vi "Main.vi"() -> ()   [LabVIEW 2025]
doc: "Use this template to build a simple state machine design pattern. Each state executes code and determines which state to transition to."
uses:
  <vilib>/Utility/miscctls.llb/LVPoint32TypeDef.ctl
  controls/State.ctl
  controls/Data.ctl
  multi.ctl
  controls/playerstatus.ctl
panel:
  in  "Boolean":bool
  out "lose":bool=TRUE
  out "win":bool=TRUE
  out "Coords":T1
  out "main tab":T2(tab) caption="Tab Control"
  in  "stop":bool
  in  "Edit entry":bool
  in  "multi entry":bool
  in  "sing entry":bool
  in  "Sp.AI entry":bool
  in  "Countdown entry":bool
  in  "Classic entry":bool
  in  "go back (sel)":bool
  in  "Size (<=25, square)":i32=3 min=3 max=25 step=1
  in  "Layers (<=64)":i32=1 min=1 max=64 step=1
  in  "Toggle barrier":bool
  in  "mapgen sw":bool
  out "multi player status":cluster{"score":i32, "name":string}[](array[cluster])
  out "score":dbl
  out "flag wrong":i32
  out "flag correct":i32
  in  "reset button":bool
  in  "page up":bool
  out "pagenum":i32
  in  "page down":bool
  out "timer":timestamp format="%<%H:%M:%S%3u>T"
  in  "go back (ingame)":bool
  out "2D Picture":picture
  in  "clean\nall\nmulti\nplayer\nand\nleave":bool
  in  "LEAVE":bool
  in  "HOST":bool
  in  "READY":bool
  out "multi player status":cluster{"score":i32, "name":string}[](array[cluster])
  out "timestart":dbl format="%_19f"
  # "map select"
  # "auto gen"
  # "load file"
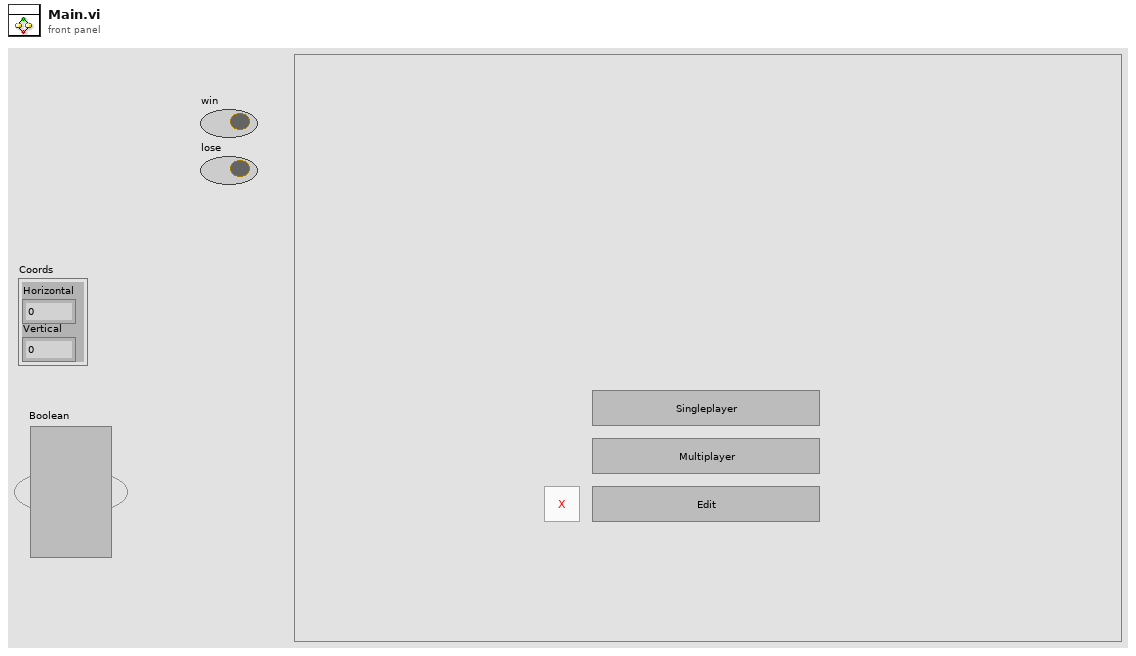
[diagram p1: front panel]
types:
  T1 = typedef "LVPoint32TypeDef.ctl" = cluster{"Horizontal":i32, "Vertical":i32}
  T2 = enum32{"menu", "select page", "sing", "multi", "multi setting"}
  T3 = typedef "Data.ctl" = cluster{"barrier":bool, "username":string, "Numeric <Replace Me>":dbl, "player mode":u16, "mode":u16, "layers":i32, "size":i32, "sec":i32}
  T4 = typedef "State.ctl" = enum16{"Initialize", "Menu", "select map", "ingame", "multi(abanden)", "edit", "Exit"}
  T5 = enum8{"Enabled", "Disabled", "Disabled and Grayed Out"}
  T6 = typedef "playerstatus.ctl" = cluster{"correct flag":i32, "wrong flag":i32, "username":string, "status":u16}
  T7 = typedef "multi.ctl" = cluster{"Array":i8[][][], "player":T6[], "layer":i32, "size":i32, "mode":u16, "sec":i32, "minecount":i32}
  T8 = cluster{"left":i16, "top":i16, "right":i16, "bottom":i16}
  T9 = typedef "LVDateTimeRec.ctl" = cluster{"fractional second":dbl, "second":i32, "minute":i32, "hour":i32, "day of month":i32, "month":i32, "year":i32, "day of week":i32, "day of year":i32, "DST":i32}
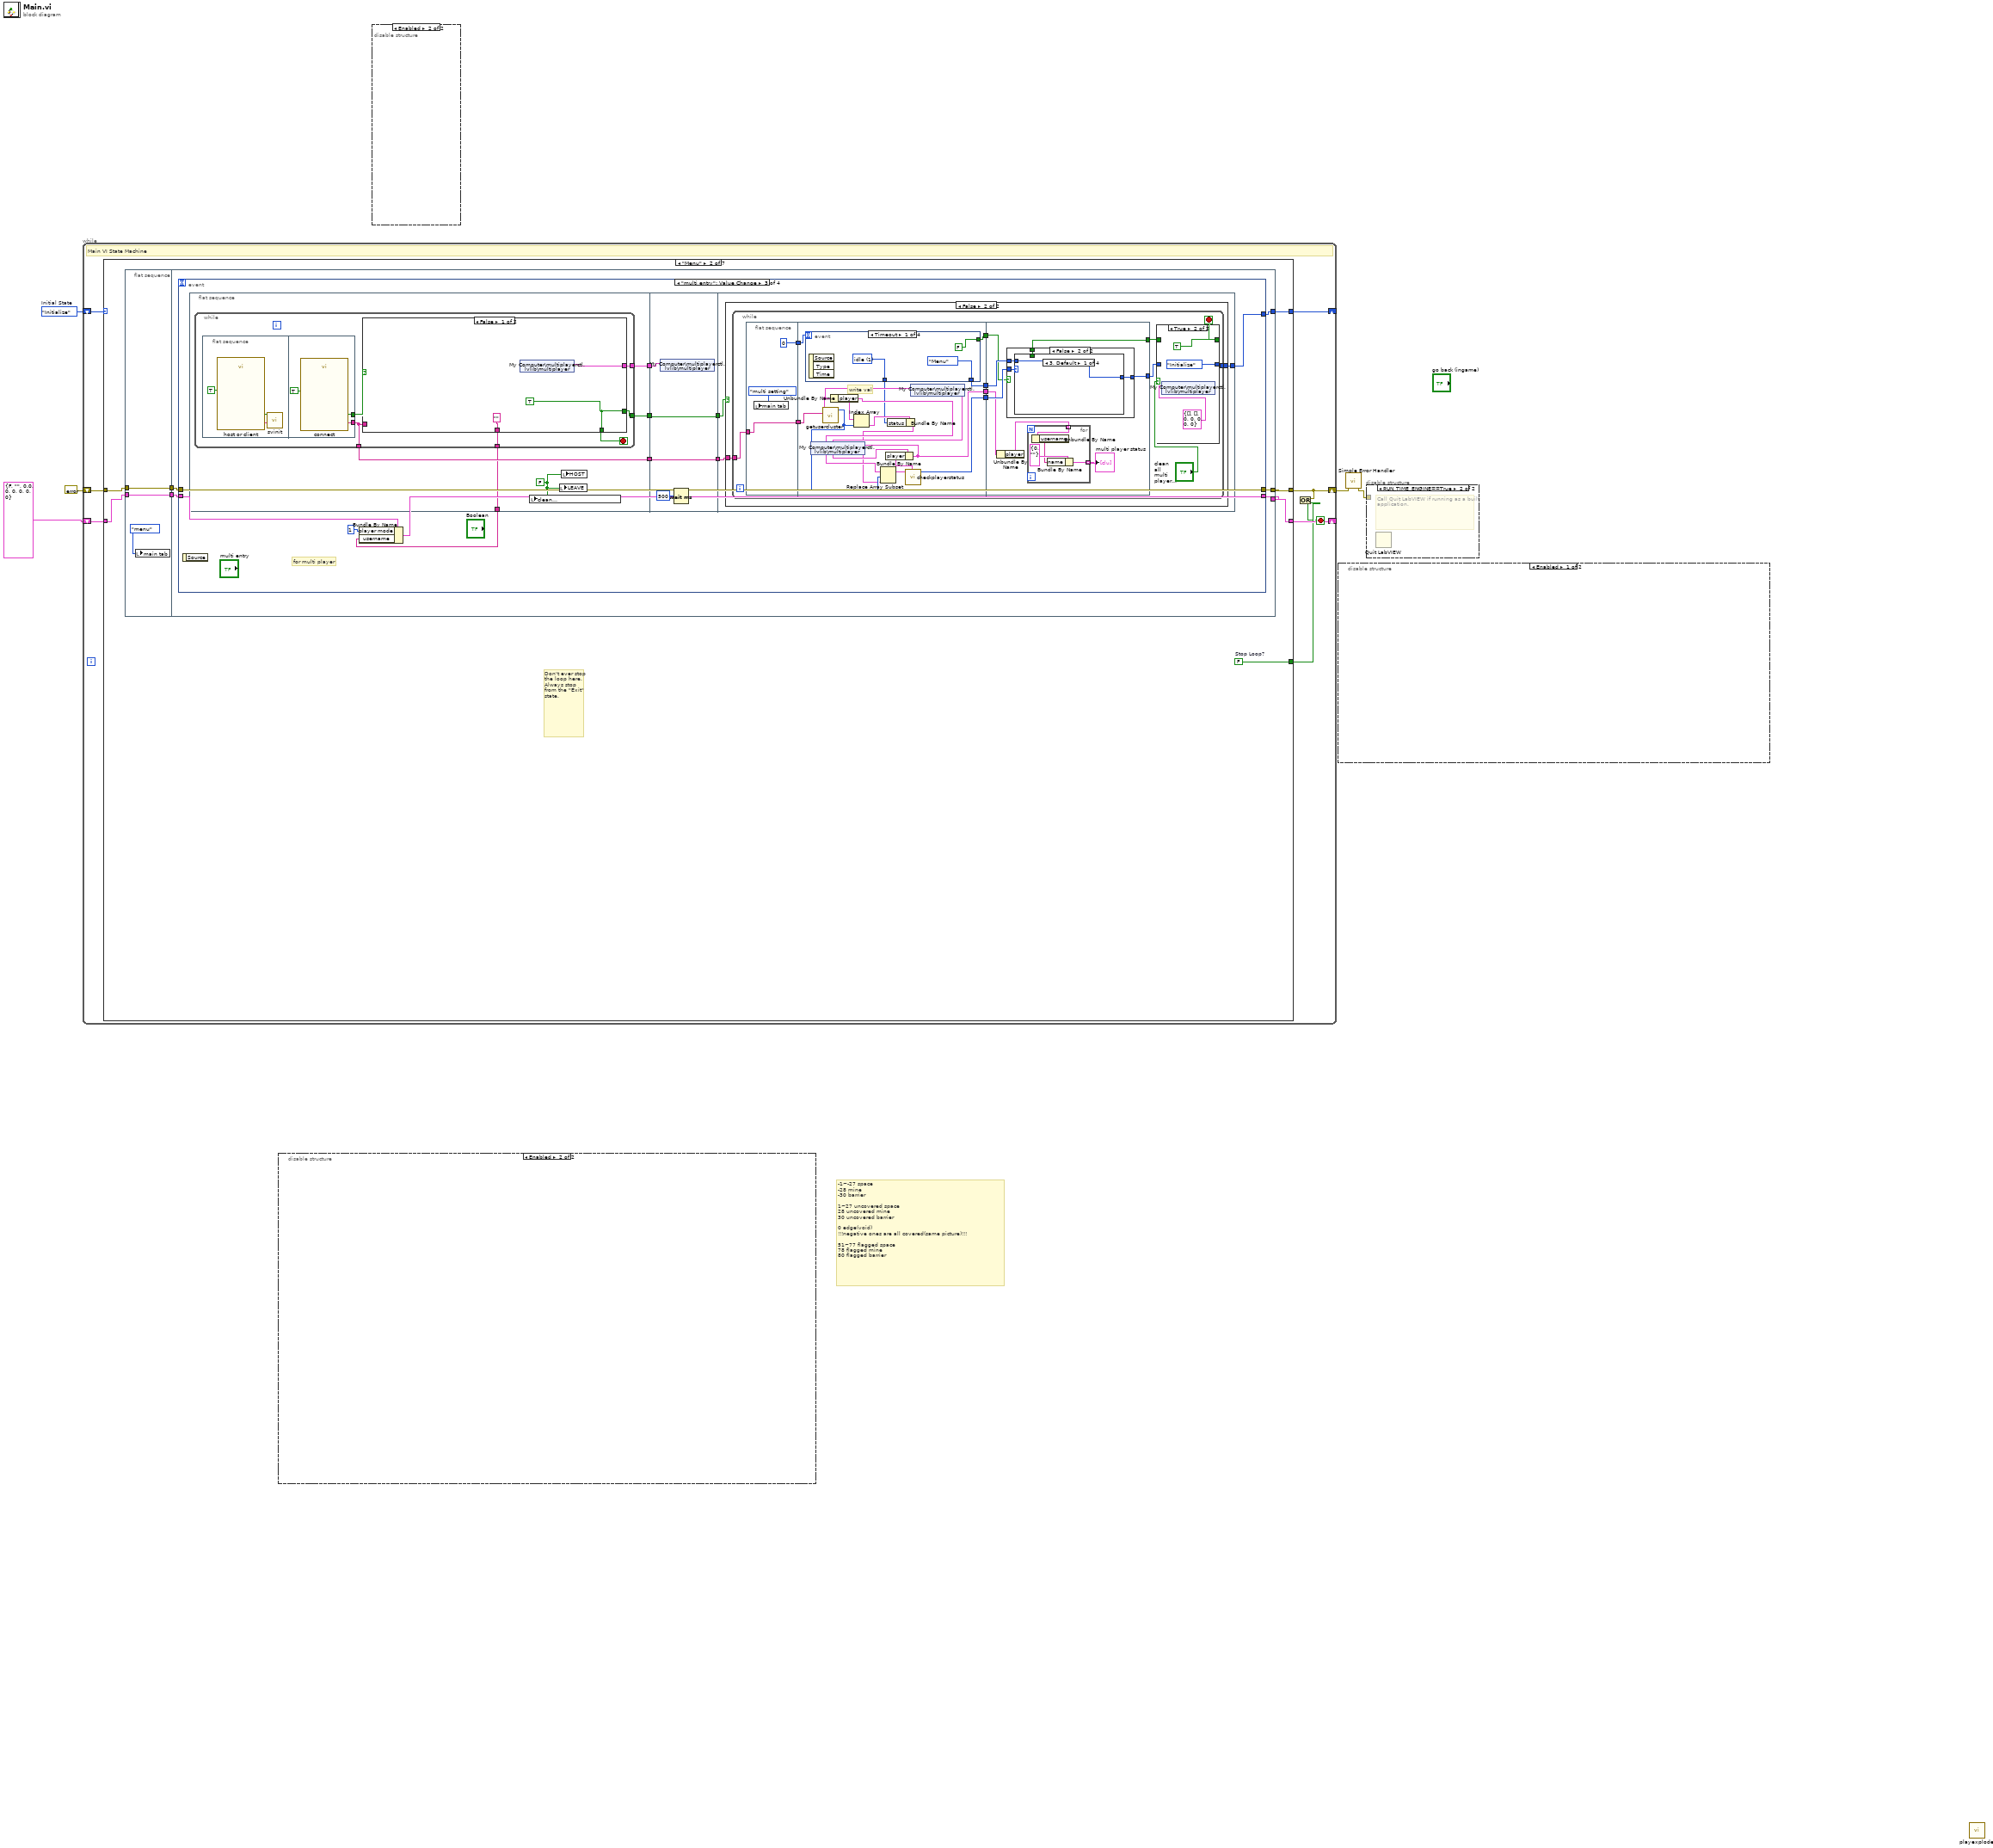
[diagram p0: block diagram]
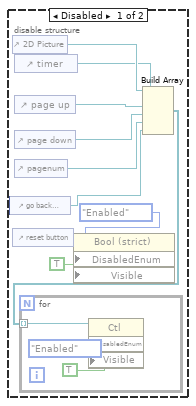
[diagram p3: hidden frame]
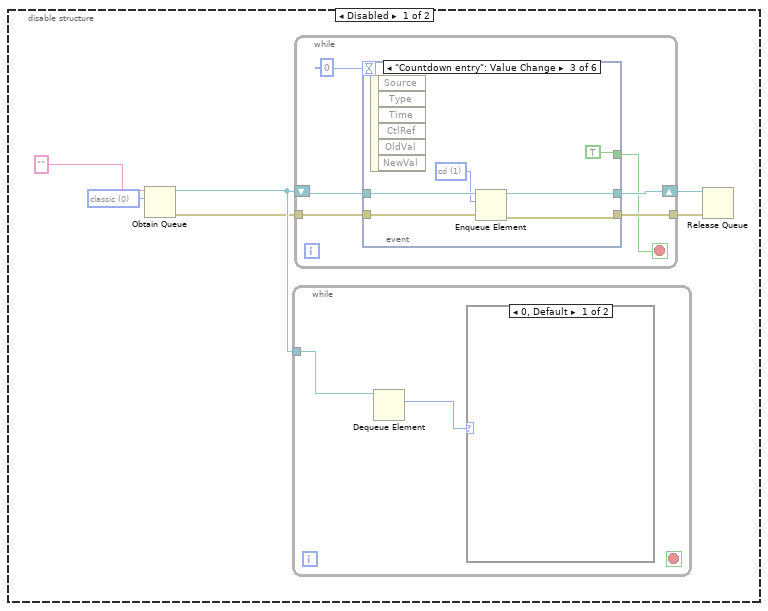
[diagram p4: hidden frame]
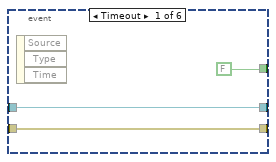
[diagram p6: hidden frame]
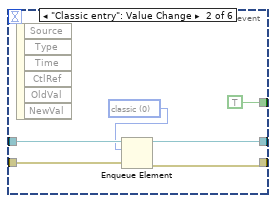
[diagram p7: hidden frame]
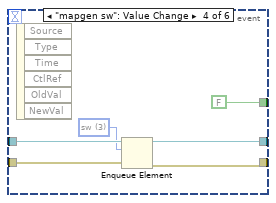
[diagram p8: hidden frame]
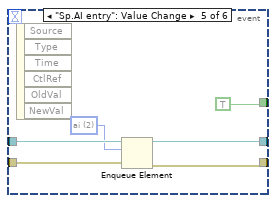
[diagram p9: hidden frame]
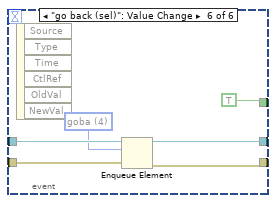
[diagram p10: hidden frame]
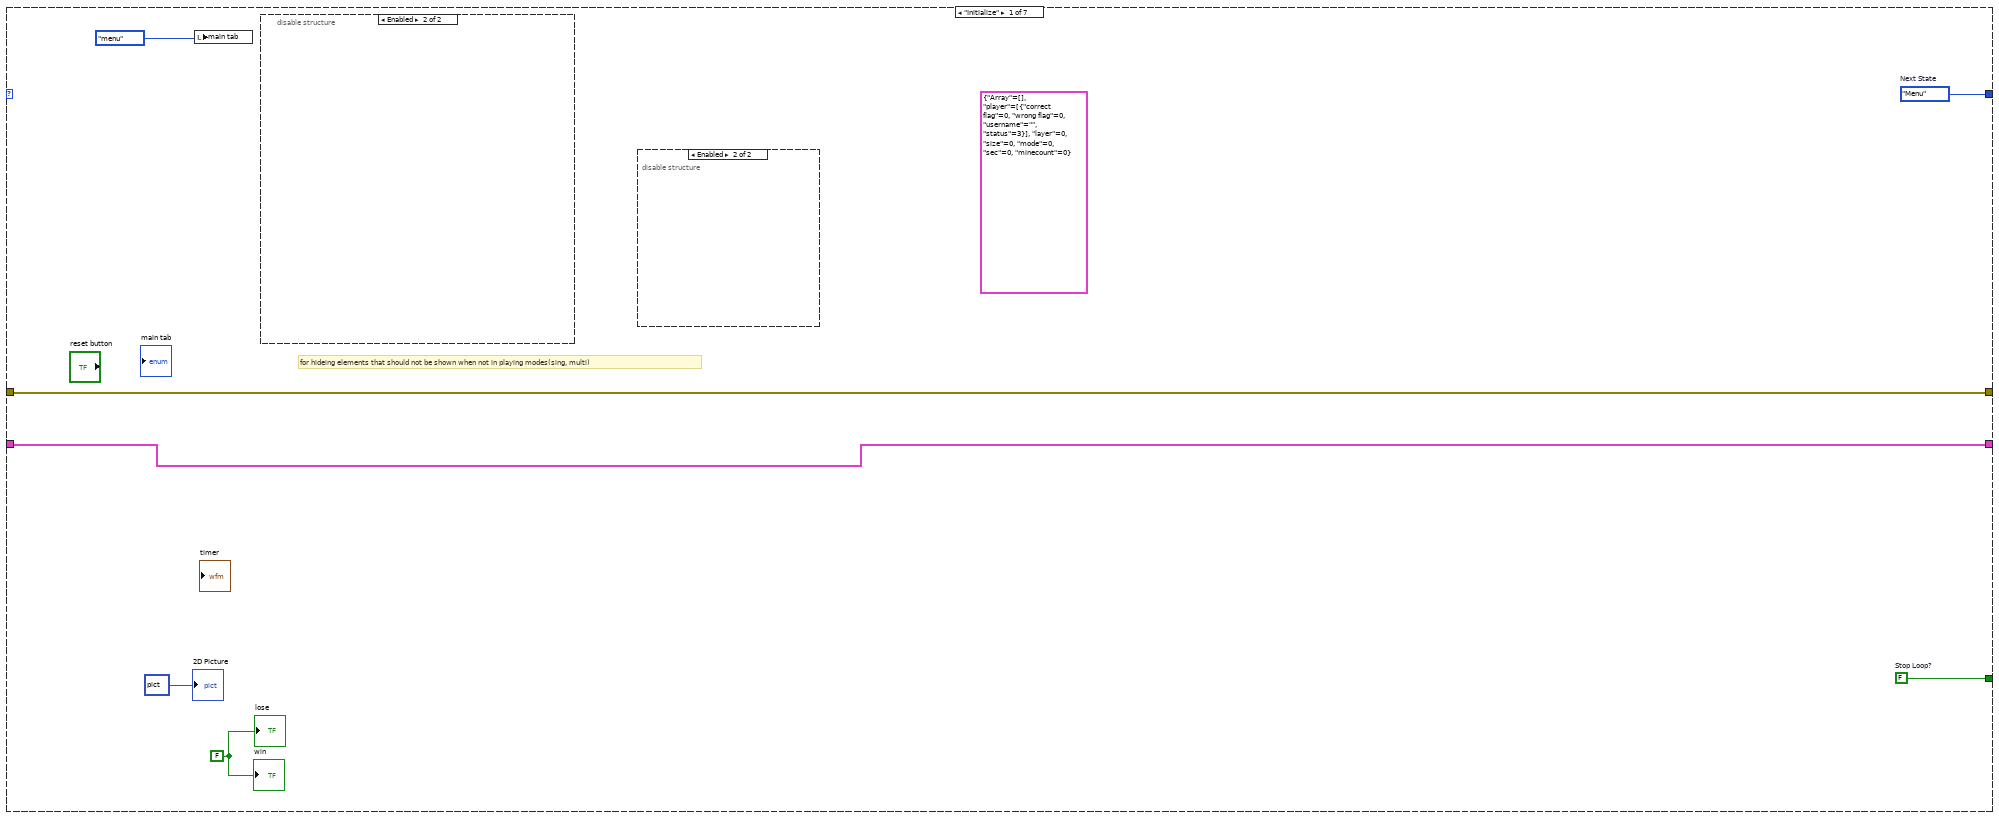
[diagram p12: hidden frame]
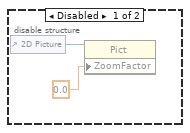
[diagram p13: hidden frame]
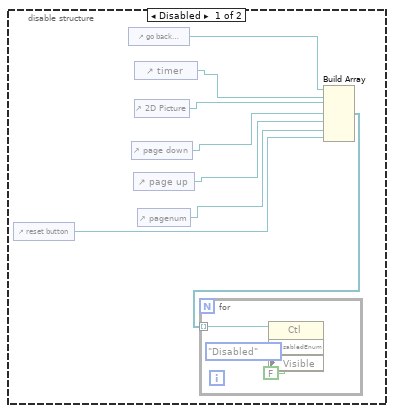
[diagram p14: hidden frame]
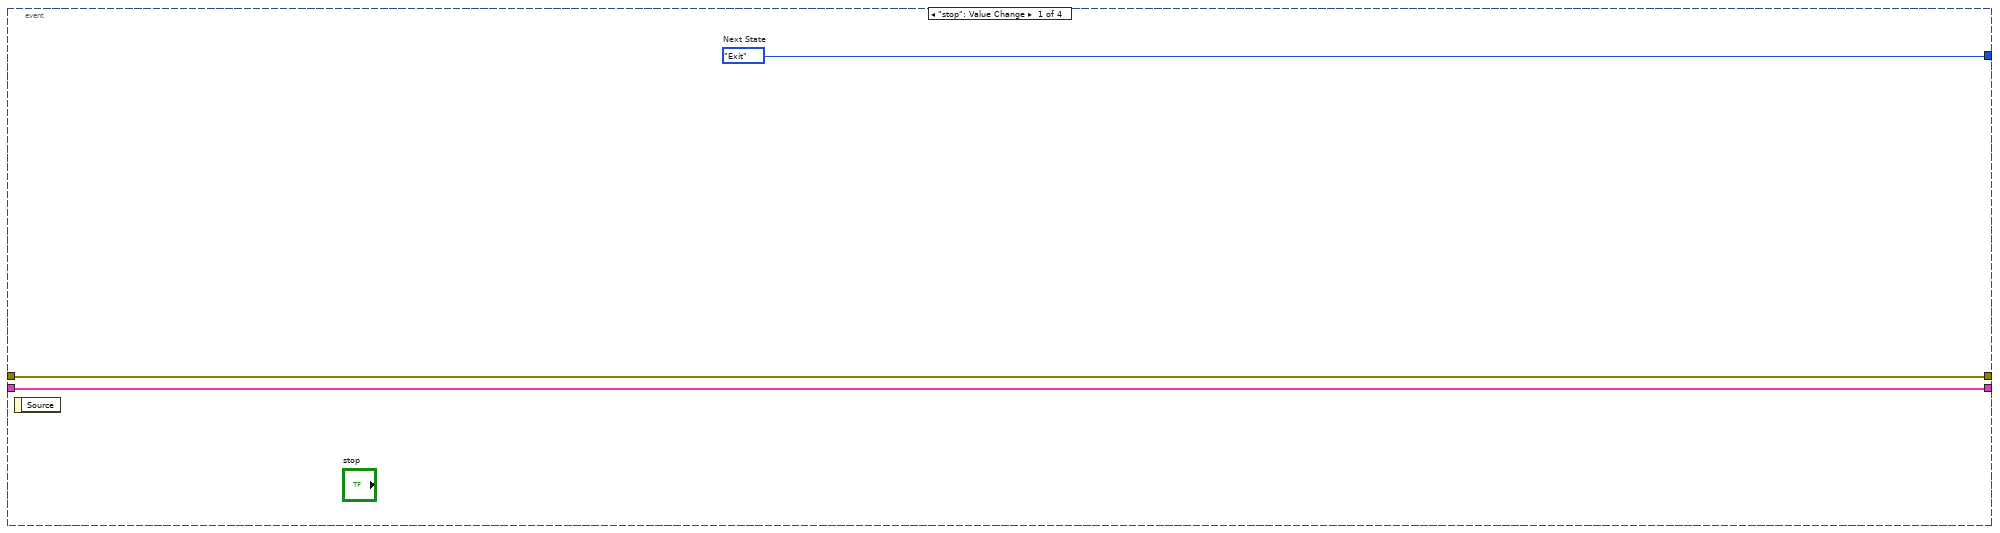
[diagram p15: hidden frame]
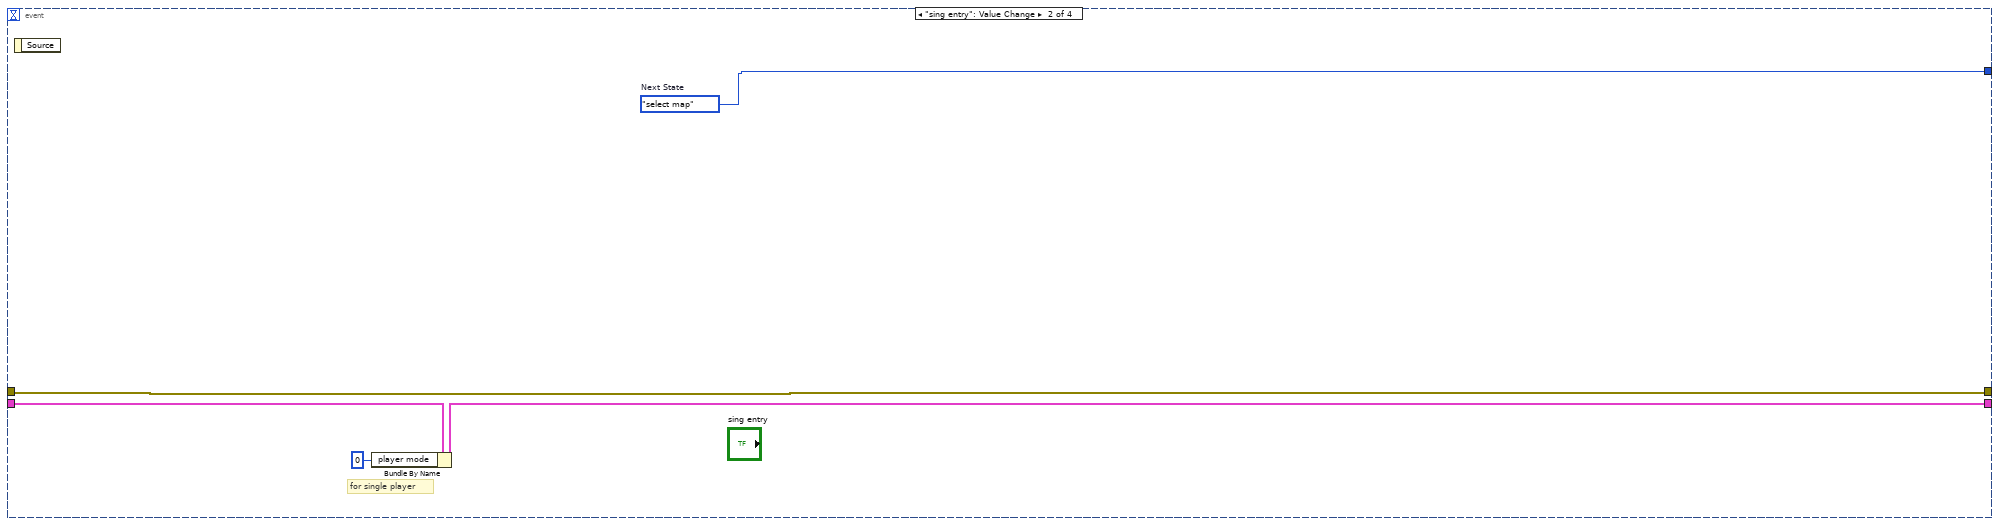
[diagram p16: hidden frame]
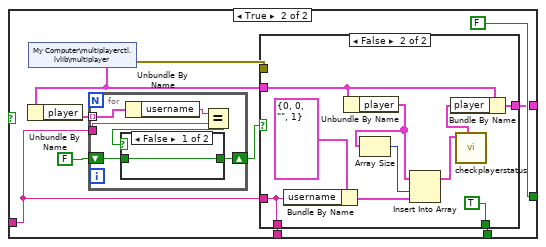
[diagram p17: hidden frame]
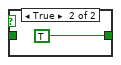
[diagram p18: hidden frame]
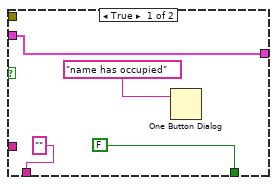
[diagram p19: hidden frame]
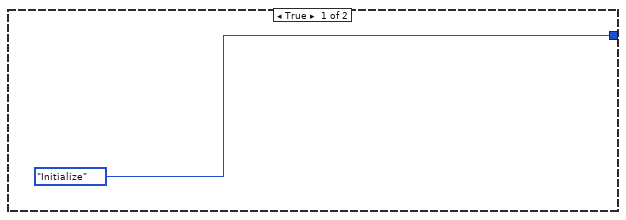
[diagram p20: hidden frame]
diagram:
  w1 = State."Initialize"  # Initial State
  # "-1~-27 space\n-28 mine\n-30 barrier\n\n1~27 uncovered space\n28 uncovered mine\n30 uncovered barrier\n\n0 edge(void)\n!!!negative ones are all covered(same picture)!!!\n\n51~77 flagged space\n78 flagged mine\n80 flagged barrier"
  n1 = while {
    shift-right: [w12] -> _
    shift-left: T3 {"barrier"=FALSE, "username"="", "Numeric <Replace Me>"=0.0, "player mode"=0, "mode"=0, "layers"=0, "size"=0, "sec"=0} ("Data") -> [w13]
    shift-right: [w8] -> w4
    shift-left: errorcluster {"status"=FALSE, "code"=0, "source"=""} ("error constant") -> [w11]
    shift-right: [w6] -> _
    shift-left: w1 -> [w7]
    stop <- w9 stop-if-true
    # "Main VI State Machine"
    n2 = case shown="\"Menu\"" w7 {
      selector: w7 -> [_ _ w204 _ _ _ _]
      tunnel: [w20 w41 w204 w209 w281 w754 w758] -> w6
      tunnel: [w19 w40 TRUE ("Stop Loop?") FALSE ("Stop Loop?") FALSE ("Stop Loop?") FALSE ("Stop Loop?") w756] -> w10
      tunnel: w13 -> [w17 w39 w207 w211 w274 w752 w757]
      tunnel: [w17 w38 w207 w212 w273 w752 w757] -> w12
      tunnel: w11 -> [w18 w37 w206 w214 w285 w751 w755]
      tunnel: [w18 w36 w206 w214 w285 w751 w755] -> w8
      frame "Initialize" {
        (unwired) T7 {"Array"=[], "player"=[{"correct flag"=0, "wrong flag"=0, "username"="", "status"=3}], "layer"=0, "size"=0, "mode"=0, "sec"=0, "minecount"=0} ("multiplayer")
        w16 = FALSE ("lose")
        w19 = FALSE  # Stop Loop?
        w20 = State."Menu"  # Next State
        # "for hideing elements that should not be shown when not in playing modes(sing, multi)"
        # "Initialize - Initialize the application."
        n3 = local write "main tab"(T2."menu" ("main tab")) -> ()
        n4 = disable-structure shown="Enabled" {
          frame Disabled {
            n5 = control-ref of="reset button"() -> (w24:refnum<vi>)
            n6 = control-ref of="go back (ingame)"() -> (w23:refnum<vi>)
            n7 = control-ref of="page down"() -> (w27:refnum<vi>)
            n8 = control-ref of="page up"() -> (w26:refnum<vi>)
            n9 = control-ref of="timer"() -> (w29:refnum<vi>)
            n10 = control-ref of="2D Picture"() -> (w28:refnum<vi>)
            n11 = control-ref of="pagenum"() -> (w25:refnum<vi>)
            n12 = Build Array(w23, w29, w28, w27, w26, w25, w24) -> (w30:refnum<vi>[])
            n13 = for {
              tunnel: w30 -> [w31] mode=indexing
              n14 = property on="Property Node" class="Ctl"(reference=w31, "DisabledEnum"=T5."Disabled" ("Disabled"), "Visible"=FALSE) -> ()  [unwired: 1 in, 2 out]
            }
          }
          frame Enabled {
          }
        }
        n15 = disable-structure shown="Enabled" {
          frame Disabled {
            n16 = control-ref of="2D Picture"() -> (w22:refnum<vi>)
            n17 = property on="Property Node" class="Pict"(reference=w22, "ZoomFactor"=sgl 0.0 ("Zoom Factor")) -> ()  [unwired: 1 in, 2 out]
          }
          frame Enabled {
          }
        }
        "win" <- w16
        "lose" <- w16
        "2D Picture" <- picture data[5B] ("2D Picture")
      }
      frame "Menu" {
        w40 = FALSE  # Stop Loop?
        # "Don't ever stop the loop here. Always stop from the \"Exit\" state."
        n18 = flat-sequence {
          tunnel: w37 -> [w43]
          tunnel: w39 -> [w44]
          tunnel: [w44] -> w35
          tunnel: [w43] -> w34
          tunnel: [w49] -> w41
          tunnel: [w45] -> w38
          tunnel: [w46] -> w36
          tunnel: w35 -> [w48]
          tunnel: w34 -> [w47]
          frame #0 {
            n19 = local write "main tab"(T2."menu" ("main tab")) -> ()
          }
          frame #1 {
            n20 = event shown="[2] \"multi entry\": Value Change" {
              selector: _ -> [_ _ _ _]
              dyn-events: _ -> [_ _ _ _]
              timeout: _ -> [_ _ _ _]
              tunnel: [w52 w56 w64 w201] -> w49
              tunnel: w48 -> [w51 w55 w66 w203]
              tunnel: [w51 w53 w65 w203] -> w45
              tunnel: w47 -> [w50 w57 w68 w202]
              tunnel: [w50 w57 w68 w202] -> w46
              event "stop": Value Change {
                w52 = State."Exit"  # Next State
                n21 = event-data() -> ()  [unwired: 1 in, 1 out]
              }
              event "sing entry": Value Change {
                w56 = State."select map"  # Next State
                # "for single player"
                n22 = event-data() -> ()  [unwired: 1 in, 1 out]
                n23 = Bundle By Name(cluster=w55, "player mode"=u16 0) -> (w53:T3)
              }
              event "multi entry": Value Change {
                # "for multi player"
                n24 = event-data() -> ()  [unwired: 1 in, 1 out]
                n25 = flat-sequence {
                  tunnel: [w73] -> w62
                  tunnel: [w72] -> w63
                  tunnel: [w71] -> w60
                  tunnel: [w70] -> w59
                  tunnel: w62 -> [w124]
                  tunnel: [w124] -> w61
                  tunnel: w60 -> [w122]
                  tunnel: w59 -> [w121]
                  tunnel: [w122] -> w58
                  tunnel: w61 -> [w127]
                  tunnel: [w126] -> w64
                  tunnel: w58 -> [w125]
                  frame #0 {
                    w69 = FALSE ("HOST")
                    n26 = while {
                      tunnel: [w78] -> w73
                      tunnel: [w77] -> w72
                      tunnel: [w75] -> w71
                      tunnel: [w74] -> w70
                      stop <- w76 stop-if-true
                      n27 = flat-sequence {
                        tunnel: [w85] -> w79
                        tunnel: [w84] -> w78
                        frame #0 {
                          n28 = call "host or client"("Enable"=TRUE) -> ("ip(client)"=w80:string, "host"=w81:bool)  [unwired: 16 in, 1 out]
                          n29 = call "svinit.vi"("ip"=w80, "host?"=w81) -> ()  [unwired: 10 in]
                        }
                        frame #1 {
                          n30 = call "connect"("Enable"=TRUE) -> ("username"=w84:string, "OK"=w85:bool)  [unwired: 16 in, 1 out]
                        }
                      }
                      n31 = case shown="False" w79 {
                        tunnel: w78 -> [_ w93]
                        tunnel: [w86 w96] -> w76
                        tunnel: ["" ("username") w92] -> w77
                        tunnel: [w86 FALSE] -> w75
                        tunnel: [w87 w89] -> w74
                        frame False {
                          w86 = TRUE
                          n32 = shared-variable "My Computer\\multiplayerctl.lvlib\\multiplayer"() -> (w87:T7)  [unwired: 1 in, 1 out]
                        }
                        frame True {
                          n33 = shared-variable "My Computer\\multiplayerctl.lvlib\\multiplayer"() -> (w98:T7, error out=w97:errorcluster)  [unwired: 1 in]
                          n34 = Unbundle By Name(w98) -> ("player"=w95:T6[])
                          n35 = for {
                            tunnel: w95 -> [w104] mode=indexing
                            tunnel: w93 -> [w102]
                            shift-right: [w100] -> w94
                            shift-left: FALSE -> [w99]
                            n36 = Unbundle By Name(w104) -> ("username"=w103:string)
                            n37 = Equal?(x=w103, y=w102) -> (x = y?=w101:bool)
                            n38 = case shown="False" w101 {
                              tunnel: [w105 TRUE] -> w100
                              tunnel: w99 -> [w105 _]
                              frame False {
                              }
                              frame True {
                              }
                            }
                          }
                          n39 = case shown="False" w94 {
                            tunnel: w98 -> [w108 w118]
                            tunnel: w97 -> [_ _]
                            tunnel: [FALSE TRUE] -> w96
                            tunnel: w93 -> [_ w115]
                            tunnel: ["" w115] -> w92
                            tunnel: [w108 w111] -> w89
                            frame True {
                              n40 = One Button Dialog(message="name has occupied") -> ()  [unwired: 1 in, 1 out]
                            }
                            frame False {
                              n41 = Bundle By Name(cluster=T6 {"correct flag"=0, "wrong flag"=0, "username"="", "status"=1} ("Cluster"), "username"=w115) -> (w116:T6)
                              n42 = Unbundle By Name(w118) -> ("player"=w117:T6[])
                              n43 = Array Size(array=w117) -> (size(s)=w114:i32)
                              n44 = Insert Into Array(array=w117, index=w114, new element=w116) -> (w113:T6[])
                              n45 = call "checkplayerstatus.vi"("player"=w113) -> ("kick leave"=w112:T6[])  [unwired: 9 in, 1 out]
                              n46 = Bundle By Name(cluster=w118, "player"=w112) -> (w111:T7)
                            }
                          }
                        }
                      }
                    }
                    n47 = local write "clean\nall\nmulti\nplayer\nand\nleave"(w69) -> ()
                    n48 = local write "LEAVE"(w69) -> ()
                    n49 = local write "HOST"(w69) -> ()
                  }
                  frame #1 {
                    n50 = shared-variable "My Computer\\multiplayerctl.lvlib\\multiplayer"(w121) -> ()  [unwired: 1 in, 1 out]
                    n51 = Wait (ms)(milliseconds to wait=u32 500) -> ()  [unwired: 1 out]
                  }
                  frame #2 {
                    n52 = case shown="False" w125 {
                      tunnel: w127 -> [_ w130]
                      tunnel: [State."Initialize" ("Initial State") w129] -> w126
                      frame True {
                      }
                      frame False {
                        n53 = while {
                          tunnel: w130 -> [w136]
                          tunnel: [w132] -> w129
                          stop <- w134 stop-if-true
                          n54 = flat-sequence {
                            tunnel: [w149] -> w142
                            tunnel: w136 -> [w149]
                            tunnel: [0] -> w141
                            tunnel: [w153] -> w139
                            tunnel: [w151] -> w138
                            tunnel: [w164] -> w140
                            tunnel: [w152] -> w137
                            tunnel: w142 -> [w156]
                            tunnel: w141 -> [w155]
                            tunnel: [w182] -> w133
                            tunnel: w140 -> [w184]
                            tunnel: w139 -> [w183]
                            tunnel: w138 -> [w178]
                            tunnel: w137 -> [w179]
                            tunnel: [w177] -> w135
                            frame #0 {
                              n55 = local write "main tab"(T2."multi setting" ("main tab")) -> ()
                            }
                            frame #1 {
                              # "write val"
                              n56 = event shown="[0] Timeout" {
                                selector: _ -> [_ _ _ _]
                                dyn-events: _ -> [_ _ _ _]
                                timeout: w155 -> [_ _ _ _]
                                tunnel: [w167 w170 w173 w176] -> w154
                                tunnel: [State."Menu" ("Initial State") State."select map" ("Initial State") State."Menu" ("Initial State") State."Initialize" ("Initial State")] -> w153
                                tunnel: [FALSE TRUE FALSE TRUE] -> w151
                                event Timeout {
                                w167 = u16 1 items=["host_ready", "idle", "host", "leaved", "ready", "playing", "lose(mine)", "lose(ot)", "win"] ("status")
                                n57 = event-data() -> ()  [unwired: 1 in, 3 out]
                                }
                                event "HOST": Value Change {
                                w170 = u16 2 items=["host_ready", "idle", "host", "leaved", "ready", "playing", "lose(mine)", "lose(ot)", "win"] ("status")
                                n58 = event-data() -> ()  [unwired: 1 in, 3 out]
                                }
                                event "READY": Value Change {
                                w173 = u16 4 items=["host_ready", "idle", "host", "leaved", "ready", "playing", "lose(mine)", "lose(ot)", "win"] ("status")
                                n59 = event-data() -> ()  [unwired: 1 in, 3 out]
                                }
                                event "LEAVE": Value Change {
                                w176 = u16 3 items=["host_ready", "idle", "host", "leaved", "ready", "playing", "lose(mine)", "lose(ot)", "win"] ("status")
                                n60 = event-data() -> ()  [unwired: 1 in, 3 out]
                                }
                              }
                              n61 = shared-variable "My Computer\\multiplayerctl.lvlib\\multiplayer"() -> (w161:T7)  [unwired: 1 in, 1 out]
                              n62 = call "getusercluster.vi"("username"=w156, "multiplayer"=w161) -> ("Numeric"=w159:i32)  [unwired: 9 in]
                              n63 = Unbundle By Name(w161) -> ("player"=w160:T6[])
                              n64 = Index Array(array=w160, index=w159) -> (element=w157:T6)
                              n65 = Bundle By Name(cluster=w157, "status"=w154) -> (w158:T6)
                              n66 = Replace Array Subset(array=w160, new element=w158, index=w159) -> (w163:T6[])
                              n67 = call "checkplayerstatus.vi"("player"=w163) -> ("Numeric"=w164:u16, "kick leave"=w162:T6[])  [unwired: 9 in]
                              n68 = Bundle By Name(cluster=w161, "player"=w162) -> (w152:T7)
                              n69 = shared-variable "My Computer\\multiplayerctl.lvlib\\multiplayer"(w152) -> ()  [unwired: 1 in, 1 out]
                            }
                            frame #2 {
                              n70 = Unbundle By Name(w179) -> ("player"=w181:T6[])
                              n71 = case shown="False" w178 {
                                selector: w178 -> [w186 _]
                                tunnel: w184 -> [_ w190]
                                tunnel: w183 -> [w185 w189]
                                tunnel: [w185 w188] -> w182
                                tunnel: [w186 w187] -> w177
                                frame True {
                                }
                                frame False {
                                n72 = case shown="3, Default" w190 {
                                tunnel: [w191 w192 State."ingame" ("Initial State") w196] -> w188
                                tunnel: w189 -> [w191 w192 _ w196]
                                tunnel: [_ _ TRUE _] -> w187
                                frame 3, Default {
                                }
                                frame 1 {
                                n73 = One Button Dialog(message="Waiting for host") -> ()  [unwired: 1 in, 1 out]
                                }
                                frame 0 {
                                }
                                frame 2 {
                                }
                                }
                                }
                              }
                              n74 = for {
                                tunnel: w181 -> [w197] mode=indexing
                                tunnel: [w198] -> w180 mode=indexing
                                n75 = Unbundle By Name(w197) -> ("username"=w199:string)
                                n76 = Bundle By Name(cluster=cluster{"score":i32, "name":string} {"score"=0, "name"=""} ("multi player status"), "name"=w199) -> (w198:cluster{"score":i32, "name":string})
                              }
                              "multi player status" <- w180
                            }
                          }
                          n77 = case shown="True" "clean\nall\nmulti\nplayer\nand\nleave" {
                            tunnel: w135 -> [w144 _]
                            tunnel: [w144 TRUE] -> w134
                            tunnel: w133 -> [w143 _]
                            tunnel: [w143 State."Initialize" ("Initial State")] -> w132
                            frame False {
                            }
                            frame True {
                              n78 = shared-variable "My Computer\\multiplayerctl.lvlib\\multiplayer"(T7 {"Array"=[], "player"=[], "layer"=0, "size"=0, "mode"=0, "sec"=0, "minecount"=0} ("Cluster")) -> ()  [unwired: 1 in, 1 out]
                            }
                          }
                        }
                      }
                    }
                  }
                }
                n79 = Bundle By Name(cluster=w66, "player mode"=u16 1, "username"=w63) -> (w65:T3)
              }
              event "Edit entry": Value Change {
                w201 = State."edit"  # Initial State
                n80 = event-data() -> ()  [unwired: 1 in, 1 out]
              }
            }
          }
        }
      }
      frame "Exit" {
      }
      frame "select map" {
        n81 = local write "main tab"(T2."select page" ("main tab")) -> ()
        n82 = Unbundle By Name(w211) -> ("player mode"=w210:u16)
        n83 = while {
          tunnel: w211 -> [w218]
          tunnel: [w217] -> w212
          tunnel: w210 -> [w216]
          tunnel: [w215] -> w209
          stop <- w219 stop-if-true
          n84 = event shown="[1] \"Classic entry\", \"Countdown entry\", \"Sp.AI entry\": Value Change" {
            selector: _ -> [_ _ _]
            dyn-events: _ -> [_ _ _]
            timeout: _ -> [_ _ _]
            tunnel: [FALSE w228 TRUE] -> w219
            tunnel: w218 -> [w223 w242 w271]
            tunnel: [w223 w243 w271] -> w217
            tunnel: w216 -> [_ w240 _]
            tunnel: [State."select map" ("(Value Not Used)") w239 State."Menu" ("(Value Not Used)")] -> w215
            event "mapgen sw": Value Change {
              # "in dev"
              n85 = event-data() -> ("NewVal"=w221:bool)  [unwired: 1 in, 5 out]
              n86 = case shown="True" w221 {
                selector: w221 -> [w225 _]
                tunnel: [w225 FALSE] -> w222
                frame False {
                }
                frame True {
                  n87 = One Button Dialog(message="developing") -> ()  [unwired: 1 in, 1 out]
                }
              }
              n88 = local write "mapgen sw"(w222) -> ()
            }
            event "Classic entry", "Countdown entry", "Sp.AI entry": Value Change {
              # "send map setting to next state"
              # "to next page"
              # "get player mode"
              # "scanning mode"
              n89 = event-data() -> ()  [unwired: 1 in, 6 out]
              n90 = case shown="True" "Classic entry" {
                tunnel: [u16 0 w268] -> w245
                frame False {
                }
                frame True {
                  w268 = u16 0 items=["classic", "countdown", "ai"]
                }
              }
              n91 = case shown="False" "Countdown entry" {
                selector: "Countdown entry" -> [w263 w265]
                tunnel: [w264 w266] -> w244
                tunnel: w245 -> [w264 _]
                tunnel: [w263 w265] -> w233
                frame False {
                }
                frame True {
                  w266 = u16 1 items=["classic", "countdown", "ai"]
                }
              }
              n92 = case shown="False" "Sp.AI entry" {
                tunnel: [w261 w262] -> w241
                tunnel: w244 -> [w261 _]
                frame False {
                }
                frame True {
                  w262 = u16 2 items=["classic", "countdown", "ai"]
                }
              }
              n93 = call "count down mode setting"("Enable"=w233) -> ("second"=w238:dbl, "minute"=w236:dbl, "GO"=w229:bool)  [unwired: 15 in, 1 out]
              n94 = Multiply(x=w236, y=60.0) -> (x*y=w237:dbl)
              n95 = Add(x=w237, y=w238) -> (x+y=w234:dbl)
              n96 = Compound Arithmetic op=OR("Classic entry", "Sp.AI entry", w229) -> (w228:bool)
              n97 = case shown="True" w228 {
                tunnel: [w251 w260] -> w243
                tunnel: w242 -> [w251 w259]
                tunnel: w241 -> [_ w254]
                tunnel: w234 -> [_ w253]
                frame False {
                }
                frame True {
                  n98 = Bundle By Name(cluster=w259, "size"="Size (<=25, square)", "layers"="Layers (<=64)", "barrier"="Toggle barrier", "mode"=w254, "sec"=w253) -> (w260:T3)
                  n99 = shared-variable "My Computer\\multiplayerctl.lvlib\\multiplayer"() -> (w257:T7)  [unwired: 1 in, 1 out]
                  n100 = Bundle By Name(cluster=w257, "layer"="Layers (<=64)", "size"="Size (<=25, square)", "mode"=w254, "sec"=w253) -> (w252:T7)
                  n101 = shared-variable "My Computer\\multiplayerctl.lvlib\\multiplayer"(w252) -> ()  [unwired: 1 in, 1 out]
                }
              }
              n102 = case shown="True" w228 {
                tunnel: w240 -> [_ w248]
                tunnel: [w246 w247] -> w239
                frame False {
                  w246 = State."select map"  # State
                }
                frame True {
                  n103 = case shown="0, Default" w248 {
                    tunnel: [State."ingame" ("(Value Not Used)") State."ingame" ("(Value Not Used)")] -> w247
                    frame 0, Default {
                    }
                    frame 1 {
                    }
                  }
                }
              }
            }
            event "go back (sel)": Value Change {
              # "go back to menu"
              n104 = event-data() -> ()  [unwired: 1 in, 6 out]
              n105 = local write "main tab"(T2."menu" ("main tab")) -> ()
            }
          }
        }
      }
      frame "ingame" {
        w281 = State."Initialize"  # Next State
        # "reset button\nin dev(12/17 done)"
        # "get map settings"
        # "User State 1 - Replace this state with functionality for your own application."
        n106 = Unbundle By Name(w274) -> ("player mode"=w275:u16)
        n107 = case shown="1" w275 {
          tunnel: w274 -> [w287 w293]
          tunnel: [w287 w290] -> w273
          frame 0, Default {
          }
          frame 1 {
            n108 = shared-variable "My Computer\\multiplayerctl.lvlib\\multiplayer"() -> (w294:T7)  [unwired: 1 in, 1 out]
            n109 = Unbundle By Name(w294) -> ("layer"=w292:i32, "size"=w291:i32, "mode"=w289:u16, "sec"=w288:i32)
            n110 = Bundle By Name(cluster=w293, "layers"=w292, "size"=w291, "mode"=w289, "sec"=w288) -> (w290:T3)
          }
        }
        n111 = Unbundle By Name(w273) -> ("layers"=w283:i32, "size"=w282:i32, "barrier"=w284:bool, "mode"=w280:u16, "sec"=w278:i32, "player mode"=w277:u16, "username"=w276:string)
        n112 = Unbundle By Name(w273) -> ("sec"=w279:i32)
        n113 = while {
          tunnel: w284 -> [w316]
          tunnel: w283 -> [w315]
          tunnel: w282 -> [w314]
          tunnel: w280 -> [w307]
          tunnel: w279 -> [w308]
          tunnel: w278 -> [w296]
          tunnel: w277 -> [w300]
          tunnel: w276 -> [w295]
          stop <- w304 stop-if-true
          w313 = FALSE ("win")
          w297 = 1
          # "2d picture \nmargin"
          # "turn on 2dpicture assist ui\ncurrent preformed in another tab"
          # "377 -30\n\n                                 1175 514"
          n114 = flat-sequence {
            tunnel: w300 -> [w660]
            tunnel: w295 -> [w661]
            tunnel: [w661] -> w302
            tunnel: [w660] -> w301
            tunnel: w314 -> [w689]
            tunnel: w315 -> [w690]
            tunnel: w316 -> [w711]
            tunnel: [w702] -> w312
            tunnel: [w701] -> w311
            tunnel: [w700] -> w309
            tunnel: [w684] -> w305
            tunnel: w302 -> [w699]
            tunnel: w301 -> [w688]
            tunnel: [w743] -> w310
            tunnel: w311 -> [w743]
            tunnel: w307 -> [w742]
            tunnel: w308 -> [w741]
            frame #0 {
              w664 = FALSE
              # "ingame"
              n115 = local write "main tab"(T2."sing" ("main tab")) -> ()
              n116 = local write "go back (ingame)"(FALSE ("go back (ingame)")) -> ()
              n117 = control-ref of="flag correct"() -> (w666:refnum<vi>)
              n118 = property on="Property Node" class="DigNum (strict)"(reference=w666, "Visible"=w664) -> ()  [unwired: 1 in, 2 out]
              n119 = control-ref of="2D Picture"() -> (w668:refnum<vi>)
              n120 = property on="Property Node" class="Pict"(reference=w668, "ZoomFactor"=sgl 1.0 ("Zoom Factor")) -> ()  [unwired: 1 in, 2 out]
              n121 = control-ref of="flag wrong"() -> (w665:refnum<vi>)
              n122 = property on="Property Node" class="DigNum (strict)"(reference=w665, "Visible"=w664) -> ()  [unwired: 1 in, 2 out]
              n123 = case shown="1" w660 {
                frame 0, Default {
                  n124 = control-ref of="multi player status"() -> (w670:refnum<vi>)
                  n125 = property on="Property Node" class="Arr (strict)"(reference=w670, "Visible"=FALSE) -> ()  [unwired: 1 in, 2 out]
                }
                frame 1 {
                  n126 = shared-variable "My Computer\\multiplayerctl.lvlib\\multiplayer"() -> (w675:T7)  [unwired: 1 in, 1 out]
                  n127 = control-ref of="multi player status"() -> (w672:refnum<vi>)
                  n128 = property on="Property Node" class="Arr (strict)"(reference=w672, "Visible"=TRUE) -> ()  [unwired: 1 in, 2 out]
                  n129 = Unbundle By Name(w675) -> ("player"=w673:T6[])
                  n130 = for {
                    tunnel: [w676] -> w674 mode=indexing
                    tunnel: w673 -> [w678] mode=indexing
                    n131 = Unbundle By Name(w678) -> ("username"=w677:string)
                    n132 = Bundle By Name(cluster=cluster{"score":i32, "name":string} {"score"=0, "name"=""} ("Array"), "name"=w677) -> (w676:cluster{"score":i32, "name":string})
                  }
                  "multi player status" <- w674
                }
              }
            }
            frame #1 {
              w681 = u16 0 items=["host_ready", "idle", "host", "leaved", "ready", "playing", "lose(mine)", "lose(ot)", "win"] ("status")
              w695 = u16 2 items=["host_ready", "idle", "host", "leaved", "ready", "playing", "lose(mine)", "lose(ot)", "win"] ("status")
              # "render once \nbefore \nevent struct."
              # "draw background"
              n133 = shared-variable "My Computer\\multiplayerctl.lvlib\\multiplayer"() -> (w698:T7)  [unwired: 1 in, 1 out]
              n134 = Unbundle By Name(w698) -> ("player"=w697:T6[])
              n135 = call "getusercluster.vi"("username"=w699, "multiplayer"=w698) -> ("Numeric"=w683:i32)  [unwired: 9 in]
              n136 = Equal To 0?(x=w688) -> (x = 0?=w694:bool)
              n137 = Index Array(array=w697, index=w683) -> (element=w682:T6)
              n138 = Bundle By Name(cluster=w682, "status"=w681) -> (w680:T6)
              n139 = Unbundle By Name(w682) -> ("status"=w696:u16)
              n140 = Not Equal To 0?(x=w688) -> (x != 0?=w686:bool)
              n141 = Equal?(x=w696, y=w695) -> (x = y?=w685:bool)
              n142 = Or(x=w694, y=w685) -> (x .or. y?=w693:bool)
              n143 = case shown="False" w693 {
                tunnel: w711 -> [_ w740]
                tunnel: [w722 w739] -> w692
                tunnel: [w721 w725] -> w691
                tunnel: [w720 w738] -> w684
                tunnel: w690 -> [w721 w725]
                tunnel: w689 -> [_ w724]
                frame False {
                  n144 = shared-variable "My Computer\\multiplayerctl.lvlib\\multiplayer"() -> (w723:T7)  [unwired: 1 in, 1 out]
                  n145 = Unbundle By Name(w723) -> ("Array"=w722:i8[][][], "minecount"=w720:i32)
                }
                frame True {
                  # "play area offset"
                  # "rng"
                  # "barrier ratio"
                  # "mine ratio"
                  # "init 3d array\n8 bit signed"
                  n146 = Decrement(x=w724) -> (x-1=w729:i32)
                  n147 = call "initarray.vi"("size"=w724, "layers"=w725) -> ("Array"=w737:i8[][][])  [unwired: 9 in]
                  n148 = Quotient & Remainder(x=w729, y=2) -> (floor(x/y)=w728:i32)  [unwired: 1 out]
                  n149 = Compound Arithmetic op=MULTIPLY(w724, w724, w725) -> (w731:i32)
                  n150 = Subtract(x=12, y=w728) -> (x-y=w727:i32)
                  n151 = Multiply(x=0.05 ("y"), y=w731) -> (x*y=w735:dbl)
                  n152 = Multiply(x=w731, y=0.02) -> (x*y=w733:dbl)
                  n153 = To Long Integer(number=w735) -> (32bit integer=w738:i32)
                  n154 = To Long Integer(number=w733) -> (32bit integer=w734:i32)
                  n155 = call "arrayrng.vi"("barrier?"=w740, "mine count"=w738, "sizeoffset"=w727, "empty array"=w737, "size"=w724, "layers"=w725, "barrier count"=w734) -> ("Array out"=w739:i8[][][])  [unwired: 4 in]
                }
              }
              n156 = And(x=w686, y=w685) -> (x .and. y?=w687:bool)
              n157 = case shown="False" w687 {
                tunnel: w692 -> [_ w718]
                tunnel: w684 -> [_ w717]
                tunnel: w683 -> [_ w714]
                tunnel: w680 -> [_ w713]
                frame False {
                }
                frame True {
                  n158 = shared-variable "My Computer\\multiplayerctl.lvlib\\multiplayer"() -> (w716:T7)  [unwired: 1 in, 1 out]
                  n159 = Unbundle By Name(w716) -> ("player"=w715:T6[])
                  n160 = Replace Array Subset(array=w715, new element=w713, index=w714) -> (w712:T6[])
                  n161 = Bundle By Name(cluster=w716, "Array"=w718, "minecount"=w717, "player"=w712) -> (w719:T7)
                  n162 = shared-variable "My Computer\\multiplayerctl.lvlib\\multiplayer"(w719) -> ()  [unwired: 1 in, 1 out]
                }
              }
              n163 = call "fillnumber.vi"("map"=w692, "size"=25 ("layers"), "layers"=w691) -> ("Array out"=w700:i8[][][])  [unwired: 8 in]
              n164 = local read "2D Picture"() -> (w709:picture)
              n165 = call "drawbg.vi"("size"=25, "2D Picture"=w709) -> ("Cluster"=w706:T8, "new picture"=w701:picture)  [unwired: 8 in]
              n166 = Unbundle By Name(w706) -> ("left"=w707:i16, "top"=w708:i16)
              n167 = Bundle("left"=w707, "top"=w708) -> (w702:cluster{"left":i16, "top":i16})  [unwired: 1 in]
              n168 = call "render.vi"("Numeric"=0, "origin"=w702, "new picture in"=w701, "map"=w700) -> ("new picture out"=w705:picture)  [unwired: 7 in]
              n169 = local write "2D Picture"(w705) -> ()
            }
            frame #2 {
              # "get x, y, z position \ndata for array"
              n170 = case shown="0, Default" w742 {
                tunnel: w741 -> [w746 _]
                frame 1 {
                  n171 = call <vilib>:"High Resolution Relative Seconds.vi"() -> ("relative seconds"=w744:dbl)
                  n172 = Seconds To Date/Time(time stamp (now)=w746, to UTC (F)=TRUE) -> (date time rec=w748:T9)
                  n173 = local write "timestart"(w744) -> ()
                  n174 = Date/Time To Seconds(2:w748) -> (0:w745:timestamp)  [unwired: 1 in]
                  n175 = local write "timer"(w745) -> ()
                }
                frame 0, Default {
                  n176 = call <vilib>:"High Resolution Relative Seconds.vi"() -> ("relative seconds"=→"timestart":dbl)
                  n177 = local write "timer"(timestamp(0 s since 1904-01-01) ("timer 2")) -> ()
                }
              }
            }
          }
          n178 = Equal?(x=u16 1, y=w300) -> (x = y?=w298:bool)
          n179 = local write "win"(w313) -> ()
          n180 = local write "lose"(w313) -> ()
          n181 = while {
            tunnel: w315 -> [w375]
            tunnel: w310 -> [w359]
            shift-right: [w374] -> _
            shift-left: w297 -> [w372]
            shift-right: [w371] -> _
            shift-left: w309 -> [w373]
            tunnel: w314 -> [w370]
            tunnel: w312 -> [w369]
            tunnel: w307 -> [w357]
            shift-right: [w366] -> _
            shift-left: 0 ("flag correct out") -> [w367]
            tunnel: w305 -> [w365]
            tunnel: [w364] -> w304
            shift-right: [w362] -> _
            shift-left: 0 ("flag correct out") -> [w363]
            tunnel: w295 -> [w356]
            tunnel: w298 -> [w355]
            stop <- w353 stop-if-true
            # "game end"
            # "one round"
            n182 = local read "lose"() -> (w361:bool)
            n183 = local read "win"() -> (w360:bool)
            n184 = call "drawwinlose.vi"("new picture in"=w359, "win"=w360, "lose"=w361) -> ("new picture out"=w358:picture)  [unwired: 8 in]
            n185 = Or(x=w361, y=w360) -> (x .or. y?=w354:bool)
            n186 = event shown="[5] Timeout" {
              selector: _ -> [_ _ _ _ _ _ _]
              dyn-events: _ -> [_ _ _ _ _ _ _]
              timeout: 10 -> [_ _ _ _ _ _ _]
              tunnel: w375 -> [w394 _ w421 _ _ _ _]
              tunnel: w369 -> [w390 _ w424 _ _ _ _]
              tunnel: w358 -> [w389 _ w425 _ _ _ w655]
              tunnel: [w382 w401 w418 w598 w608 w617 w652] -> w374
              tunnel: w373 -> [w381 _ w420 w599 w606 w618 w653]
              tunnel: w372 -> [w383 w401 w419 w598 w608 w617 w652]
              tunnel: [w381 i8[][][] [] ("Array out") w422 w599 w606 w618 w653] -> w371
              tunnel: w370 -> [_ _ w423 _ _ _ _]
              tunnel: [FALSE w395 _ FALSE FALSE FALSE w654] -> w353
              tunnel: w354 -> [w377 _ w417 _ _ w615 _]
              tunnel: w367 -> [w379 w400 w409 w601 w604 w610 w651]
              tunnel: [w379 w400 w411 w601 w604 w610 w651] -> w366
              tunnel: w365 -> [_ _ w415 _ _ w614 _]
              tunnel: [_ TRUE _ _ _ _ _] -> w364
              tunnel: [w376 w398 w410 w600 w603 w609 w650] -> w362
              tunnel: w363 -> [w376 w398 w408 w600 w603 w609 w650]
              tunnel: w356 -> [_ w396 w414 _ _ w612 _]
              tunnel: w355 -> [_ w397 w413 w592 _ w611 w646]
              tunnel: w357 -> [_ _ w412 _ _ _ _]
              event "page up", "page down": Value Change {
                # "re-render after current page change"
                # "page control"
                n187 = event-data() -> ()  [unwired: 1 in, 6 out]
                n188 = Increment(x=w383) -> (x+1=w393:i32)
                n189 = Select(t=w393, s="page up", f=w383) -> (s? t:f=w392:i32)
                n190 = Decrement(x=w392) -> (x-1=w391:i32)
                n191 = Select(t=w391, s="page down", f=w392) -> (s? t:f=w387:i32)
                n192 = In Range and Coerce(upper limit=w394, x=w387, lower limit=1) -> (coerced(x)=w382:i32)  [unwired: 1 out]
                n193 = Decrement(x=w382) -> (x-1=w388:i32)
                n194 = call "render.vi"("game end?"=w377, "Numeric"=w388, "origin"=w390, "new picture in"=w389, "map"=w381) -> ("new picture out"=w380:picture)  [unwired: 6 in]
                n195 = local write "2D Picture"(w380) -> ()
                n196 = local write "pagenum"(w382) -> ()
              }
              event "go back (ingame)": Value Change {
                w395 = TRUE
                n197 = event-data() -> ()  [unwired: 1 in, 6 out]
                n198 = case shown="True" w397 {
                  selector: w397 -> [_ w407]
                  tunnel: w396 -> [_ w404]
                  frame False {
                  }
                  frame True {
                    w403 = u16 3 items=["host_ready", "idle", "host", "leaved", "ready", "playing", "lose(mine)", "lose(ot)", "win"] ("status")
                    n199 = shared-variable "My Computer\\multiplayerctl.lvlib\\multiplayer"() -> (w405:T7)  [unwired: 1 in, 1 out]
                    n200 = call "userstatusRW.vi"("write?"=w407, "username"=w404, "status"=w403, "Cluster in"=w405) -> ("Cluster out"=w406:T7)  [unwired: 6 in, 1 out]
                    n201 = shared-variable "My Computer\\multiplayerctl.lvlib\\multiplayer"(w406) -> ()  [unwired: 1 in, 1 out]
                  }
                }
                n202 = local write "lose"(w395) -> ()
              }
              event "2D Picture": Mouse Down {
                # "flc"
                # "flw"
                # "mode"
                # "mode"
                # "layers"
                # "page"
                n203 = event-data() -> ("Coords"=w426:T1, "Button"=w416:u16)  [unwired: 1 in, 6 out]
                n204 = case shown="False" w417 {
                  tunnel: w426 -> [_ w444]
                  tunnel: w425 -> [_ w452]
                  tunnel: w424 -> [_ w446]
                  tunnel: w423 -> [_ w451]
                  tunnel: [w430 w450] -> w422
                  tunnel: w421 -> [_ w449]
                  tunnel: w420 -> [w430 w431]
                  tunnel: w419 -> [w429 w448]
                  tunnel: [w429 w447] -> w418
                  tunnel: w416 -> [_ w440]
                  tunnel: w415 -> [_ w439]
                  tunnel: w414 -> [_ w438]
                  tunnel: w413 -> [_ w437]
                  tunnel: w412 -> [_ w436]
                  tunnel: w409 -> [w428 w435]
                  tunnel: [w427 w434] -> w410
                  tunnel: [w428 w433] -> w411
                  tunnel: w408 -> [w427 w432]
                  frame True {
                    # "game end"
                  }
                  frame False {
                    w443 = T1 {"Horizontal"=580, "Vertical"=-5} ("upper limit")
                    n205 = Add(x=500, y=w443) -> (x+y=w441:T1)
                    n206 = In Range and Coerce(upper limit=w441, x=w444, lower limit=w443) -> (In Range?=w445:bool)  [unwired: 1 out]
                    n207 = case shown="True" w445 {
                      tunnel: w452 -> [_ w479]
                      tunnel: w446 -> [_ w478]
                      tunnel: w451 -> [_ w465]
                      tunnel: [w456 w477] -> w450
                      tunnel: w449 -> [_ w472]
                      tunnel: w431 -> [w456 w459]
                      tunnel: w448 -> [w455 w476]
                      tunnel: [w455 w475] -> w447
                      tunnel: w444 -> [_ w471]
                      tunnel: w446 -> [_ w470]
                      tunnel: w440 -> [_ w474]
                      tunnel: w439 -> [_ w473]
                      tunnel: w438 -> [_ w467]
                      tunnel: w437 -> [_ w466]
                      tunnel: w436 -> [_ w464]
                      tunnel: w435 -> [w454 w461]
                      tunnel: [w453 w458] -> w434
                      tunnel: w432 -> [w453 w460]
                      tunnel: [w454 w457] -> w433
                      frame False {
                      }
                      frame True {
                        w463 = u16 2 items=["classic", "countdown", "ai"] ("mode")
                        n208 = Equal?(x=w464, y=w463) -> (x = y?=w462:bool)
                        n209 = call "click.vi"("page"=w472, "Coords"=w471, "Cluster"=w470, "size"=w465) -> ("y"=w469:i32, "x"=w468:i32)  [unwired: 6 in]
                        n210 = while {
                          tunnel: w479 -> [w481]
                          tunnel: w478 -> [w509]
                          tunnel: w473 -> [w507]
                          tunnel: w469 -> [w496]
                          tunnel: w468 -> [w497]
                          tunnel: w467 -> [w506]
                          tunnel: w466 -> [w505]
                          tunnel: w462 -> [w494]
                          shift-right: [w480] -> w477
                          shift-left: w459 -> [w504]
                          shift-right: [w485] -> _
                          shift-left: _ -> [w495]
                          shift-right: [w490] -> _
                          shift-left: w474 -> [w491]
                          shift-right: [w488] -> w457
                          shift-left: w461 -> [w489]
                          shift-right: [w486] -> w458
                          shift-left: w460 -> [w487]
                          shift-right: [w492] -> w475
                          shift-left: w476 -> [w508]
                          i -> [w503]
                          stop <- w482 stop-if-true
                          # "w/l\nchk\naft.\nassign"
                          # "ai chk"
                          n211 = Unbundle(w495) -> ("y"=w499:i32, "x"=w498:i32)  [unwired: 2 out]
                          n212 = Equal To 0?(x=w503) -> (x = 0?=w502:bool)
                          n213 = case shown="False" w502 {
                            tunnel: w497 -> [_ w538]
                            tunnel: w496 -> [_ w539]
                            tunnel: [w537 w539] -> w501
                            tunnel: [w536 w538] -> w500
                            tunnel: w499 -> [w537 _]
                            tunnel: w498 -> [w536 _]
                            frame False {
                            }
                            frame True {
                            }
                          }
                          n214 = disable-structure shown="Disabled" {
                            frame Disabled {
                              n215 = Wait (ms)(milliseconds to wait=u32 1) -> ()  [unwired: 1 out]
                            }
                            frame Enabled {
                            }
                          }
                          n216 = flat-sequence {
                            tunnel: w508 -> [w570]
                            tunnel: [w570] -> w512
                            tunnel: w491 -> [w564]
                            tunnel: w507 -> [w561]
                            tunnel: w501 -> [w563]
                            tunnel: w500 -> [w562]
                            tunnel: [w558] -> w511
                            tunnel: w506 -> [w557]
                            tunnel: w505 -> [w555]
                            tunnel: w494 -> [w554]
                            tunnel: [w552] -> w510
                            tunnel: [w540] -> w485
                            tunnel: w504 -> [w551]
                            tunnel: w489 -> [w550]
                            tunnel: [w549] -> w488
                            tunnel: w487 -> [w548]
                            tunnel: [w547] -> w486
                            tunnel: w509 -> [w590]
                            tunnel: w481 -> [w589]
                            tunnel: [w588] -> w480
                            tunnel: w512 -> [w587]
                            tunnel: [w587] -> w493
                            tunnel: w511 -> [w584]
                            tunnel: w510 -> [w588]
                            frame #0 {
                              w559 = u16 6 items=["host_ready", "idle", "host", "leaved", "ready", "playing", "lose(mine)", "lose(ot)", "win"] ("status")
                              # "uncoverspace"
                              # "uncover clicked"
                              n217 = Decrement(x=w570) -> (x-1=w572:i32)
                              n218 = Index Array(array=w551, index (dim 0)=w572, index (dim 1)=w563, index (dim 2)=w562) -> (element=w569:i8)
                              n219 = call "manageclick.vi"("in"=w569, "total mine"=w561, "Button"=w564, "flag wrong in"=w550, "flag correct in"=w548) -> ("out"=w573:i8, "lose"=w546:bool, "flag wrong out"=w549:i32, "flag correct out"=w547:i32, "win1"=w545:bool)  [unwired: 6 in]
                              n220 = shared-variable "My Computer\\multiplayerctl.lvlib\\multiplayer"() -> (w560:T7)  [unwired: 1 in, 1 out]
                              n221 = Replace Array Subset(array=w551, new element=w573, index (dim 0)=w572, index (dim 1)=w563, index (dim 2)=w562) -> (w571:i8[][][])
                              n222 = call "uncoverspace.vi"("input array"=w571, "j"=w562, "i"=w563, "k"=w572) -> ("win?"=w568:i32, "output array"=w553:i8[][][], "win2"=w544:i32)  [unwired: 5 in]
                              n223 = Equal?(x=w544, y=1) -> (x = y?=w542:bool)
                              n224 = And(x=w542, y=w545) -> (x .and. y?=w541:bool)
                              n225 = Equal?(x=w568, y=1) -> (x = y?=w565:bool)
                              n226 = Or(x=w541, y=w565) -> (x .or. y?=w566:bool)
                              n227 = local write "win"(w566) -> ()
                              n228 = local write "lose"(w546) -> ()
                              n229 = And(x=w546, y=w555) -> (x .and. y?=w556:bool)
                              n230 = call "userstatusRW.vi"("write?"=w556, "username"=w557, "status"=w559, "Cluster in"=w560) -> ("Cluster out"=w558:T7)  [unwired: 6 in, 1 out]
                              n231 = case shown="True" w554 {
                                tunnel: w553 -> [w574 w576]
                                tunnel: [w574 w576] -> w552
                                tunnel: [_ w577] -> w540
                                frame False {
                                }
                                frame True {
                                n232 = call "dllpathselect.vi"() -> ("appended path"=w575:path)  [unwired: 11 in]
                                n233 = dll-call lib="C:/Users/daimapi/Desktop/programmar/minesweeper/c_code/main.dll" fn="ai"(path in=w575, "arg1"=w576) -> ("z"=w581:i32, "y"=w580:i32, "x"=w579:i32, "action"=w578:i32)  [unwired: 8 in, 2 out]
                                n234 = Bundle("z"=w581, "y"=w580, "x"=w579, "action"=w578) -> (w577:cluster{"z":i32, "y":i32, "x":i32, "action":i32})  [unwired: 1 in]
                                }
                              }
                            }
                            frame #1 {
                              # "render and show"
                              n235 = Decrement(x=w587) -> (x-1=w591:i32)
                              n236 = local read "lose"() -> (w583:bool)
                              n237 = local read "win"() -> (w585:bool)
                              n238 = shared-variable "My Computer\\multiplayerctl.lvlib\\multiplayer"(w584) -> ()  [unwired: 1 in, 1 out]
                              n239 = call "render.vi"("game end?"=w583, "Numeric"=w591, "origin"=w590, "new picture in"=w589, "map"=w588) -> ("new picture out"=w582:picture)  [unwired: 6 in]
                              n240 = local write "pagenum"(w587) -> ()
                              n241 = call "drawwinlose.vi"("new picture in"=w582, "win"=w585, "lose"=w583) -> ("new picture out"=w586:picture)  [unwired: 8 in]
                              n242 = local write "2D Picture"(w586) -> ()
                              n243 = call "playexplode.vi"("2D Picture"=w582, "lose"=w583) -> ()  [unwired: 10 in]
                            }
                          }
                          n244 = Unbundle By Name(w485) -> ("z"=w484:i32, "action"=w483:i32)
                          n245 = case shown="True" w494 {
                            tunnel: w484 -> [_ w525]
                            tunnel: w493 -> [w516 w521]
                            tunnel: [w516 w524] -> w492
                            tunnel: w483 -> [_ w523]
                            tunnel: w491 -> [w515 w522]
                            tunnel: [w515 w526] -> w490
                            tunnel: [TRUE w517] -> w482
                            frame False {
                            }
                            frame True {
                              n246 = case shown="0, Default" w523 {
                                selector: w523 -> [_ w532 w535]
                                tunnel: [w527 w532 w535] -> w526
                                tunnel: [TRUE _ _] -> w518
                                tunnel: w525 -> [_ w531 w534]
                                tunnel: [w528 w530 w533] -> w524
                                tunnel: w521 -> [w528 _ _]
                                tunnel: w522 -> [w527 _ _]
                                frame 0, Default {
                                # "no\nact"
                                }
                                frame 1 {
                                n247 = Increment(x=w531) -> (x+1=w530:i32)
                                }
                                frame 3 {
                                n248 = Increment(x=w534) -> (x+1=w533:i32)
                                }
                              }
                              n249 = local read "lose"() -> (w519:bool)
                              n250 = local read "win"() -> (w520:bool)
                              n251 = Compound Arithmetic op=OR(w518, w519, w520) -> (w517:bool)
                            }
                          }
                        }
                      }
                    }
                  }
                }
              }
              event "win", "lose": Value Change {
                w596 = u16 8 items=["host_ready", "idle", "host", "leaved", "ready", "playing", "lose(mine)", "lose(ot)", "win"] ("status")
                # "this will trigger only if manul change val"
                n252 = event-data() -> ()  [unwired: 1 in, 6 out]
                n253 = shared-variable "My Computer\\multiplayerctl.lvlib\\multiplayer"() -> (w597:T7)  [unwired: 1 in, 1 out]
                n254 = local read "win"() -> (w594:bool)
                n255 = And(x=w594, y=w592) -> (x .and. y?=w593:bool)
                n256 = call "userstatusRW.vi"("write?"=w593, "status"=w596, "Cluster in"=w597) -> ("Cluster out"=w595:T7)  [unwired: 7 in, 1 out]
                n257 = shared-variable "My Computer\\multiplayerctl.lvlib\\multiplayer"(w595) -> ()  [unwired: 1 in, 1 out]
              }
              event "2D Picture": Mouse Move {
                # "for debug"
                n258 = event-data() -> ("Coords"=→"Coords":T1)  [unwired: 1 in, 4 out]
              }
              event Timeout {
                n259 = event-data() -> ()  [unwired: 1 in, 3 out]
                n260 = case shown="False" w615 {
                  tunnel: w609 -> [_ w640]
                  tunnel: w610 -> [_ w641]
                  tunnel: w614 -> [_ w642]
                  tunnel: [0.0 w634] -> w613
                  frame False {
                    w630 = FALSE
                    n261 = control-ref of="flag wrong"() -> (w631:refnum<vi>)
                    n262 = control-ref of="flag correct"() -> (w632:refnum<vi>)
                    n263 = property on="Property Node" class="DigNum (strict)"(reference=w631, "Visible"=w630) -> ()  [unwired: 1 in, 2 out]
                    n264 = property on="Property Node" class="DigNum (strict)"(reference=w632, "Visible"=w630) -> ()  [unwired: 1 in, 2 out]
                  }
                  frame True {
                    w637 = TRUE
                    n265 = control-ref of="flag correct"() -> (w639:refnum<vi>)
                    n266 = control-ref of="flag wrong"() -> (w638:refnum<vi>)
                    n267 = Subtract(x=w640, y=w641) -> (x-y=w643:i32)
                    n268 = local read "win"() -> (w636:bool)
                    n269 = property on="Property Node" class="DigNum (strict)"(reference=w639, "Visible"=w637) -> ()  [unwired: 1 in, 2 out]
                    n270 = property on="Property Node" class="DigNum (strict)"(reference=w638, "Visible"=w637) -> ()  [unwired: 1 in, 2 out]
                    n271 = Divide(x=w643, y=w642) -> (x/y=w635:dbl)
                    n272 = case shown="False" w636 {
                      tunnel: w635 -> [w644 _]
                      tunnel: [w644 1.0] -> w634
                      frame False {
                      }
                      frame True {
                      }
                    }
                  }
                }
                "score" <- w613
                n273 = case shown="True" w611 {
                  tunnel: w612 -> [_ w629]
                  tunnel: w610 -> [_ w627]
                  tunnel: w609 -> [_ w626]
                  frame False {
                  }
                  frame True {
                    # "kick leaved"
                    n274 = shared-variable "My Computer\\multiplayerctl.lvlib\\multiplayer"() -> (w622:T7)  [unwired: 1 in, 1 out]
                    n275 = call "getusercluster.vi"("username"=w629, "multiplayer"=w622) -> ("Numeric"=w625:i32)  [unwired: 9 in]
                    n276 = Unbundle By Name(w622) -> ("player"=w623:T6[])
                    n277 = Index Array(array=w623, index=w625) -> (element=w628:T6)
                    n278 = Bundle By Name(cluster=w628, "correct flag"=w627, "wrong flag"=w626) -> (w624:T6)
                    n279 = Replace Array Subset(array=w623, new element=w624, index=w625) -> (w620:T6[])
                    n280 = call "checkplayerstatus.vi"("player"=w620) -> ("kick leave"=w619:T6[])  [unwired: 9 in, 1 out]
                    n281 = Bundle By Name(cluster=w622, "player"=w619) -> (w621:T7)
                    n282 = shared-variable "My Computer\\multiplayerctl.lvlib\\multiplayer"(w621) -> ()  [unwired: 1 in, 1 out]
                  }
                }
                "flag wrong" <- w610
                "flag correct" <- w609
              }
              event "reset button": Value Change {
                # "end round"
                n283 = event-data() -> ("NewVal"=w648:bool)  [unwired: 1 in, 5 out]
                n284 = Not(x=w646) -> (.not. x?=w647:bool)
                n285 = And(x=w648, y=w647) -> (x .and. y?=w649:bool)
                n286 = case shown="True" w649 {
                  tunnel: w655 -> [_ _]
                  tunnel: [FALSE TRUE] -> w654
                  frame False {
                  }
                  frame True {
                    n287 = call "Empty Picture"() -> ("empty picture"=w658:picture)
                    n288 = local write "2D Picture"(w658) -> ()
                    n289 = local write "lose"(TRUE) -> ()
                  }
                }
              }
            }
          }
          n290 = while {
            tunnel: w296 -> [w324]
            tunnel: w307 -> [w323]
            tunnel: w295 -> [w322]
            tunnel: w298 -> [w321]
            stop <- w317 stop-if-true
            n291 = case shown="0, Default" w323 {
              tunnel: [w325 w341] -> w320
              tunnel: w324 -> [_ w339]
              tunnel: w322 -> [_ w332]
              tunnel: w321 -> [_ w331]
              frame 0, Default {
                n292 = local read "timestart"() -> (w328:dbl)
                n293 = call <vilib>:"High Resolution Relative Seconds.vi"() -> ("relative seconds"=w330:dbl)
                n294 = Subtract(x=w330, y=w328) -> (x-y=w329:dbl)
                n295 = Seconds To Date/Time(time stamp (now)=w329, to UTC (F)=TRUE) -> (date time rec=w327:T9)
                n296 = Date/Time To Seconds(2:w327) -> (0:w325:timestamp)  [unwired: 1 in]
              }
              frame 1 {
                n297 = local read "timestart"() -> (w334:dbl)
                n298 = call <vilib>:"High Resolution Relative Seconds.vi"() -> ("relative seconds"=w333:dbl)
                n299 = Subtract(x=w333, y=w334) -> (x-y=w340:dbl)
                n300 = Subtract(x=w339, y=w340) -> (x-y=w338:dbl)
                n301 = local read "2D Picture"() -> (w335:picture)
                n302 = Less Or Equal?(x=w338, y=0.0) -> (x <= y?=w336:bool)
                n303 = Seconds To Date/Time(time stamp (now)=w338, to UTC (F)=TRUE) -> (date time rec=w343:T9)
                n304 = Date/Time To Seconds(2:w343) -> (0:w341:timestamp)  [unwired: 1 in]
                n305 = case shown="True" w336 {
                  selector: w336 -> [_ w350]
                  tunnel: w335 -> [_ w352]
                  tunnel: w331 -> [_ w349]
                  tunnel: w332 -> [_ w345]
                  frame False {
                  }
                  frame True {
                    w344 = u16 7 items=["host_ready", "idle", "host", "leaved", "ready", "playing", "lose(mine)", "lose(ot)", "win"] ("status")
                    n306 = local write "lose"(w350) -> ()
                    n307 = And(x=w349, y=w350) -> (x .and. y?=w348:bool)
                    n308 = call "drawwinlose.vi"("new picture in"=w352, "lose"=w350) -> ("new picture out"=w351:picture)  [unwired: 9 in]
                    n309 = shared-variable "My Computer\\multiplayerctl.lvlib\\multiplayer"() -> (w346:T7)  [unwired: 1 in, 1 out]
                    n310 = local write "2D Picture"(w351) -> ()
                    n311 = call "userstatusRW.vi"("write?"=w348, "username"=w345, "status"=w344, "Cluster in"=w346) -> ("Cluster out"=w347:T7)  [unwired: 6 in, 1 out]
                    n312 = shared-variable "My Computer\\multiplayerctl.lvlib\\multiplayer"(w347) -> ()  [unwired: 1 in, 1 out]
                  }
                }
              }
            }
            n313 = local read "lose"() -> (w318:bool)
            n314 = local read "win"() -> (w319:bool)
            n315 = Compound Arithmetic op=OR(w319, w318) -> (w317:bool)
            n316 = local write "timer"(w320) -> ()
          }
          "pagenum" <- w297
        }
      }
      frame "multi(abanden)" {
        w754 = State."Initialize"  # Next State
        # "in dev"
        # "User State 2 - Replace this state with functionality for your own application."
      }
      frame "edit" {
        w756 = TRUE  # Stop Loop?
        w758 = State."Exit"  # (Value Not Used)
        # "The state value is not used here since this is the last iteration of the state machine loop."
        # "Exit - Exit the application."
      }
    }
    n317 = Or(x=w8, y=w10) -> (x .or. y?=w9:bool)
  }
  n318 = disable-structure shown="Enabled" {
    frame Disabled {
      w759 = u16 0 items=["classic", "cd", "ai", "sw", "goba"]
      n319 = Obtain Queue(name (unnamed)="", element data type=w759) -> (queue out=w763:refnum<queue>, error out=w761:errorcluster)  [unwired: 3 in, 1 out]
      n320 = while {
        tunnel: w763 -> [w766]
        stop <- _ stop-if-true
        n321 = Dequeue Element(queue=w766) -> (element=w765:u16)  [unwired: 2 in, 3 out]
        n322 = case shown="0, Default" w765 {
          frame 0, Default {
          }
          frame 1 {
          }
        }
      }
      n323 = while {
        shift-right: [w771] -> w762
        shift-left: w763 -> [w772]
        tunnel: w761 -> [w770]
        tunnel: [w769] -> w760
        stop <- w767 stop-if-true
        n324 = event shown="[2] \"Countdown entry\": Value Change" {
          selector: _ -> [_ _ _ _ _ _]
          dyn-events: _ -> [_ _ _ _ _ _]
          timeout: 0 ("Numeric") -> [_ _ _ _ _ _]
          tunnel: [w775 w781 w787 w793 w799 w805] -> w771
          tunnel: w772 -> [w775 w779 w785 w791 w797 w803]
          tunnel: w770 -> [w774 w778 w784 w790 w796 w802]
          tunnel: [w774 w780 w786 w792 w798 w804] -> w769
          tunnel: [FALSE TRUE TRUE FALSE TRUE TRUE] -> w767
          event Timeout {
            n325 = event-data() -> ()  [unwired: 1 in, 3 out]
          }
          event "Classic entry": Value Change {
            w776 = u16 0 items=["classic", "cd", "ai", "sw", "goba"]
            n326 = event-data() -> ()  [unwired: 1 in, 6 out]
            n327 = Enqueue Element(queue=w779, element=w776, error in (no error)=w778) -> (queue out=w781:refnum<queue>, error out=w780:errorcluster)  [unwired: 1 in, 1 out]
          }
          event "Countdown entry": Value Change {
            w782 = u16 1 items=["classic", "cd", "ai", "sw", "goba"]
            n328 = event-data() -> ()  [unwired: 1 in, 6 out]
            n329 = Enqueue Element(queue=w785, element=w782, error in (no error)=w784) -> (queue out=w787:refnum<queue>, error out=w786:errorcluster)  [unwired: 1 in, 1 out]
          }
          event "mapgen sw": Value Change {
            w789 = u16 3 items=["single", "muti", "ai", "sw", "goba"]
            n330 = event-data() -> ()  [unwired: 1 in, 6 out]
            n331 = Enqueue Element(queue=w791, element=w789, error in (no error)=w790) -> (queue out=w793:refnum<queue>, error out=w792:errorcluster)  [unwired: 1 in, 1 out]
          }
          event "Sp.AI entry": Value Change {
            w795 = u16 2 items=["single", "muti", "ai", "sw", "goba"]
            n332 = event-data() -> ()  [unwired: 1 in, 6 out]
            n333 = Enqueue Element(queue=w797, element=w795, error in (no error)=w796) -> (queue out=w799:refnum<queue>, error out=w798:errorcluster)  [unwired: 1 in, 1 out]
          }
          event "go back (sel)": Value Change {
            w801 = u16 4 items=["single", "muti", "ai", "sw", "goba"]
            n334 = event-data() -> ()  [unwired: 1 in, 6 out]
            n335 = Enqueue Element(queue=w803, element=w801, error in (no error)=w802) -> (queue out=w805:refnum<queue>, error out=w804:errorcluster)  [unwired: 1 in, 1 out]
          }
        }
      }
      n336 = Release Queue(queue=w762, error in (no error)=w760) -> ()  [unwired: 1 in, 3 out]
    }
    frame Enabled {
    }
  }
  n337 = disable-structure shown="Enabled" {
    frame Disabled {
      n338 = control-ref of="go back (ingame)"() -> (w806:refnum<vi>)
      n339 = control-ref of="2D Picture"() -> (w814:refnum<vi>)
      n340 = control-ref of="reset button"() -> (w809:refnum<vi>)
      n341 = control-ref of="timer"() -> (w813:refnum<vi>)
      n342 = control-ref of="page up"() -> (w812:refnum<vi>)
      n343 = control-ref of="page down"() -> (w811:refnum<vi>)
      n344 = control-ref of="pagenum"() -> (w810:refnum<vi>)
      n345 = property on="Property Node" class="Bool (strict)"(reference=w809, "DisabledEnum"=T5."Enabled" ("Disabled"), "Visible"=TRUE) -> ()  [unwired: 1 in, 2 out]
      n346 = Build Array(w814, w813, w812, w811, w810, w806) -> (w815:refnum<vi>[])
      n347 = for {
        tunnel: w815 -> [w816] mode=indexing
        n348 = property on="Property Node" class="Ctl"(reference=w816, "DisabledEnum"=T5."Enabled" ("Disabled"), "Visible"=TRUE) -> ()  [unwired: 1 in, 2 out]
      }
    }
    frame Enabled {
    }
  }
  n349 = disable-structure shown="Enabled" {
    frame Enabled {
    }
    frame Disabled {
    }
  }
  n350 = call <vilib>:"Simple Error Handler.vi"("error in (no error)"=w4) -> ("error out"=w3:errorcluster)  [unwired: 4 in, 4 out]
  n351 = disable-structure shown="RUN_TIME_ENGINE==True" {
    disable-tunnel: w3 -> [_ _]
    frame condition #0 (active) {
    }
    frame condition #1 {
      # "Call Quit LabVIEW if running as a built application."
      n352 = Quit LabVIEW() -> ()  [unwired: 1 in]
    }
  }
  n353 = call "playexplode.vi"() -> ()  [unwired: 12 in]
